vi "tune samples.vi"(7 "compensation":T1, 9 "input valid":bool, 10 "channels in":T1) -> (1 "output valid":bool, 2 "channels out":T1)   [LabVIEW 2020]
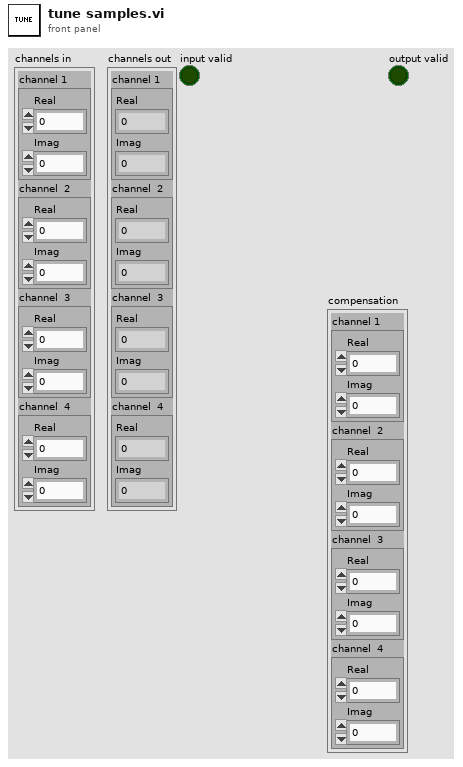
[diagram p1: front panel]
types:
  T1 = cluster{"channel 1 ":cluster{"Real":fxp<+/-,16,3>, "Imag":fxp<+/-,16,3>}, "channel  2":cluster{"Real":fxp<+/-,16,3>, "Imag":fxp<+/-,16,3>}, "channel  3":cluster{"Real":fxp<+/-,16,3>, "Imag":fxp<+/-,16,3>}, "channel  4":cluster{"Real":fxp<+/-,16,3>, "Imag":fxp<+/-,16,3>}}
  T2 = cluster{"Real":fxp<+/-,16,3>, "Imag":fxp<+/-,16,3>}
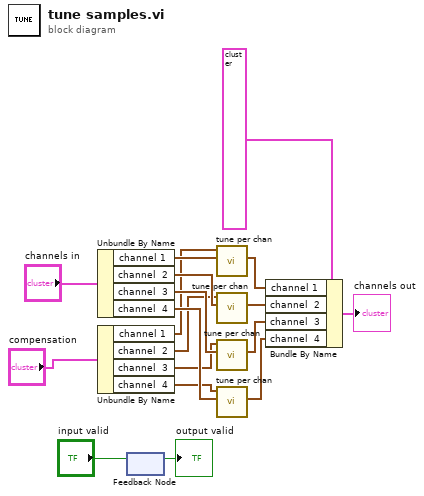
[diagram p0: block diagram]
diagram:
  n1 = Unbundle By Name("channels in") -> ("channel 1"=w15:T2, "channel  2"=w10:T2, "channel  3"=w9:T2, "channel  4"=w8:T2)
  n2 = Unbundle By Name("compensation") -> ("channel 1"=w3:T2, "channel  2"=w4:T2, "channel  3"=w1:T2, "channel  4"=w2:T2)
  n3 = feedback-in #1("input valid") -> ()
  n4 = feedback #1() -> (→"output valid":bool)  [unwired: 1 in]
  n5 = call "tune per chan.vi"("channel in"=w15, "compensation"=w3) -> ("channel out"=w14:T2)  [unwired: 9 in]
  n6 = call "tune per chan.vi"("channel in"=w10, "compensation"=w4) -> ("channel out"=w7:T2)  [unwired: 9 in]
  n7 = call "tune per chan.vi"("channel in"=w9, "compensation"=w1) -> ("channel out"=w6:T2)  [unwired: 9 in]
  n8 = call "tune per chan.vi"("channel in"=w8, "compensation"=w2) -> ("channel out"=w5:T2)  [unwired: 9 in]
  n9 = Bundle By Name(cluster=T1 {"channel 1 "={"Real"=0.0, "Imag"=0.0}, "channel  2"={"Real"=0.0, "Imag"=0.0}, "channel  3"={"Real"=0.0, "Imag"=0.0}, "channel  4"={"Real"=0.0, "Imag"=0.0}} ("channels out"), "channel 1"=w14, "channel  2"=w7, "channel  3"=w6, "channel  4"=w5) -> (→"channels out":T1)
